vi "TestExec.Load Route List.vi"(9 "Station Name":string, 11 "Route List File":path) -> (3 "Route List":string[](array[string]))   [LabVIEW 2018]
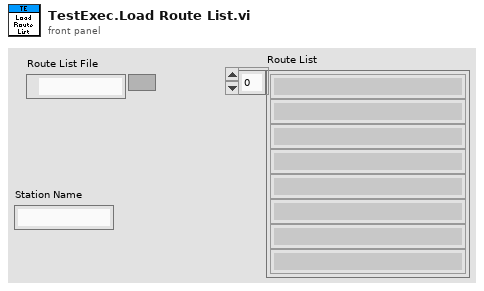
[diagram p1: front panel]
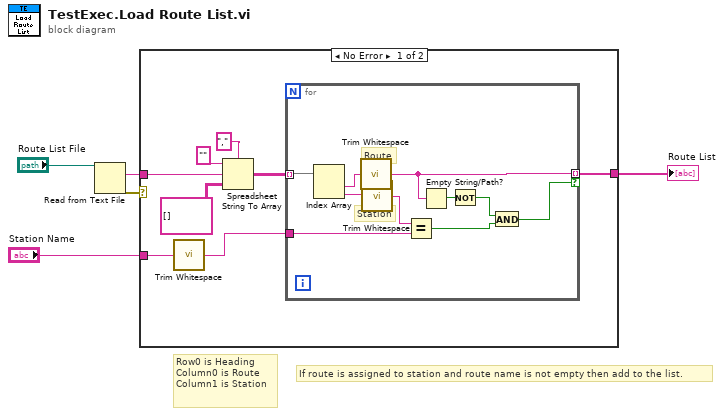
[diagram p0: block diagram]
diagram:
  # "If route is assigned to station and route name is not empty then add to the list."
  # "Row0 is Heading\nColumn0 is Route\nColumn1 is Station"
  n1 = Read from Text File(file (use dialog)="Route List File") -> (text=w5:string, error out=w3:errorcluster)  [unwired: 3 in, 2 out]
  n2 = case shown="No Error" w3 {
    tunnel: w5 -> [w13 _]
    tunnel: "Station Name" -> [w8 _]
    tunnel: [w6 _] -> w1
    frame No Error {
      n3 = call <vilib>:"Trim Whitespace.vi"("string"=w8) -> ("trimmed string"=w7:string)  [unwired: 1 in]
      n4 = Spreadsheet String To Array(delimiter (Tab)=",", format string="", spreadsheet string=w13, array type (2D Dbl)=string[][] []) -> (array=w9:string[][])
      n5 = for {
        tunnel: w9 -> [w21] mode=indexing
        tunnel: [w23] -> w6 mode=indexing if=w14
        tunnel: w7 -> [w17]
        # "Station"
        # "Route"
        n6 = Index Array(array=w21) -> (element #1=w20:string, element #2=w19:string)  [unwired: 2 in]
        n7 = call <vilib>:"Trim Whitespace.vi"("string"=w20) -> ("trimmed string"=w23:string)  [unwired: 1 in]
        n8 = call <vilib>:"Trim Whitespace.vi"("string"=w19) -> ("trimmed string"=w18:string)  [unwired: 1 in]
        n9 = Equal?(x=w18, y=w17) -> (x = y?=w15:bool)
        n10 = Empty String/Path?(string/path=w23) -> (empty?=w22:bool)
        n11 = Not(x=w22) -> (.not. x?=w16:bool)
        n12 = And(x=w16, y=w15) -> (x .and. y?=w14:bool)
      }
    }
    frame Error {
    }
  }
  "Route List" <- w1
